vi "C to F.vi"(10 "Value [°C]":dbl) -> (2 "Value [°F]":dbl)   [LabVIEW 2013, in "Dual Mode Thermometer.lvclass"]
doc: "Copyright (c) 2016 Sze Howe Koh\nThis code is licensed under the MIT license"
uses:
  Dual Mode Thermometer.lvclass
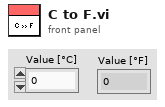
[diagram p1: front panel]
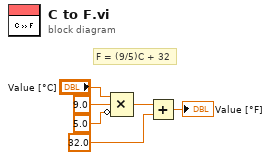
[diagram p0: block diagram]
diagram:
  # "F = (9/5)C + 32"
  n1 = Compound Arithmetic op=MULTIPLY("Value [°C]", 9.0 ("value"), invert 5.0 ("value")) -> (w2:dbl)
  n2 = Add(x=w2, y=32.0) -> (x+y=→"Value [°F]":dbl)
